vi "Reset layer template selection.vi"(7 "Force reset? (T)":bool=TRUE, 8 "error in (no error)":errorcluster, 11 "Data in":T1={"Class"={"Ants"=refnum, "Layer"=refnum, "Templates"=refnum, "Icon"=refnum, "Glyph"=refnum, "Settings"=refnum, "Tools"=refnum}, "Ref"={"Add Layer"=refnum, "Remove Layer"=refnum, "Line Text"=[], "Body Text Spec"=refnum, "DNL_Font"=refnum, "glyph path str"=refnum, "templates path str"=refnum, "Arrow Up"=refnum, "Arrow Down"=refnum, "IE VI Ref"=refnum, "Glyphs tree"=refnum, "Templates tree"=refnum, "Layer Icon Text"=refnum, "Layer Template"=refnum, "Clipboard"=refnum, "BW icon in"=refnum, "Color icon in"=refnum, "Layer Clust"=refnum, "Body Text"=refnum, "DNL_Framework Templates"=refnum, "Search Templates"=refnum, "TextMarker"=refnum, "Tab Control"=refnum, "Search Glyphs"=refnum, "Line Color"=refnum, "DNL_Glyphs []"=refnum, "Fill Color"=refnum, "Tools"=refnum, "Glyphs tree"=refnum, "Icon"=refnum, "Preview"=refnum, "Ants"=refnum, "Terminals"=refnum, "menu reference"=refnum, "LayerNames"=[], "GlyphLoadAnimation"=refnum, "TemplateLoadAnimation"=refnum, "refreshGlyphs"=refnum, "refreshTemplates"=refnum}, "Support"={"AntsRect"={"left"=0, "top"=0, "right"=0, "bottom"=0}, "Mouse Move Coords"={"Horizontal"=0, "Vertical"=0}, "Mouse Down Coords"={"Horizontal"=0, "Vertical"=0}, "Temp Coord"={"Horizontal"=0, "Vertical"=0}, "Action"=enum."Default", "Edge Color"=4914962, "Fill Color"=16860, "Mouse Down?"=FALSE, "Draft Mode?"=FALSE, "Temp Icon"=bytes[3102], "CTRL Pressed"=FALSE, "Move Selection?"=FALSE, "AntsRect Orig"={"left"=0, "top"=0, "right"=0, "bottom"=0}, "Text"="", "TM Set?"=FALSE, "Mouse inside icon?"=FALSE, "Tool (old value)"=0, "Pencil Move Color"=0, "Swap Colors?"=FALSE, "Shift pressed?"=FALSE}}) -> (0 "error out":errorcluster, 2 "Active Data []":i32[](array[numeric]), 3 "Data out":T1={"Class"={"Ants"=refnum, "Layer"=refnum, "Templates"=refnum, "Icon"=refnum, "Glyph"=refnum, "Settings"=refnum, "Tools"=refnum}, "Ref"={"Add Layer"=refnum, "Remove Layer"=refnum, "Line Text"=[], "Body Text Spec"=refnum, "DNL_Font"=refnum, "glyph path str"=refnum, "templates path str"=refnum, "Arrow Up"=refnum, "Arrow Down"=refnum, "IE VI Ref"=refnum, "Glyphs tree"=refnum, "Templates tree"=refnum, "Layer Icon Text"=refnum, "Layer Template"=refnum, "Clipboard"=refnum, "BW icon in"=refnum, "Color icon in"=refnum, "Layer Clust"=refnum, "Body Text"=refnum, "DNL_Framework Templates"=refnum, "Search Templates"=refnum, "TextMarker"=refnum, "Tab Control"=refnum, "Search Glyphs"=refnum, "Line Color"=refnum, "DNL_Glyphs []"=refnum, "Fill Color"=refnum, "Tools"=refnum, "Glyphs tree"=refnum, "Icon"=refnum, "Preview"=refnum, "Ants"=refnum, "Terminals"=refnum, "menu reference"=refnum, "LayerNames"=[], "GlyphLoadAnimation"=refnum, "TemplateLoadAnimation"=refnum, "refreshGlyphs"=refnum, "refreshTemplates"=refnum}, "Support"={"AntsRect"={"left"=0, "top"=0, "right"=0, "bottom"=0}, "Mouse Move Coords"={"Horizontal"=0, "Vertical"=0}, "Mouse Down Coords"={"Horizontal"=0, "Vertical"=0}, "Temp Coord"={"Horizontal"=0, "Vertical"=0}, "Action"=enum."Default", "Edge Color"=4914962, "Fill Color"=16860, "Mouse Down?"=FALSE, "Draft Mode?"=FALSE, "Temp Icon"=bytes[3102], "CTRL Pressed"=FALSE, "Move Selection?"=FALSE, "AntsRect Orig"={"left"=0, "top"=0, "right"=0, "bottom"=0}, "Text"="", "TM Set?"=FALSE, "Mouse inside icon?"=FALSE, "Tool (old value)"=0, "Pencil Move Color"=0, "Swap Colors?"=FALSE, "Shift pressed?"=FALSE}}, 5 "Layers selected?":bool)   [LabVIEW 2021]
uses:
  Controls/IE Data.ctl
  Class/Ants/Ants.lvclass
  Class/FakedArray/FakedArray.lvclass
  vi.lib/LabVIEW Icon API/lv_icon/Classes/Icon/Icon.lvclass
  Class/Icon Library/Glyph.lvclass
  Class/Settings/Settings.lvclass
  Class/Tools/Tools Paint.lvclass
  Controls/IE Classes.ctl
  Controls/References Cluster.ctl
  Controls/SupportClass.ctl
  <vilib>/Utility/miscctls.llb/LVPoint32TypeDef.ctl
  Controls/SupportClass_Action.ctl
  vi.lib/LabVIEW Icon API/lv_icon/Controls/IEColor.ctl
  Global Variables/Data.vi
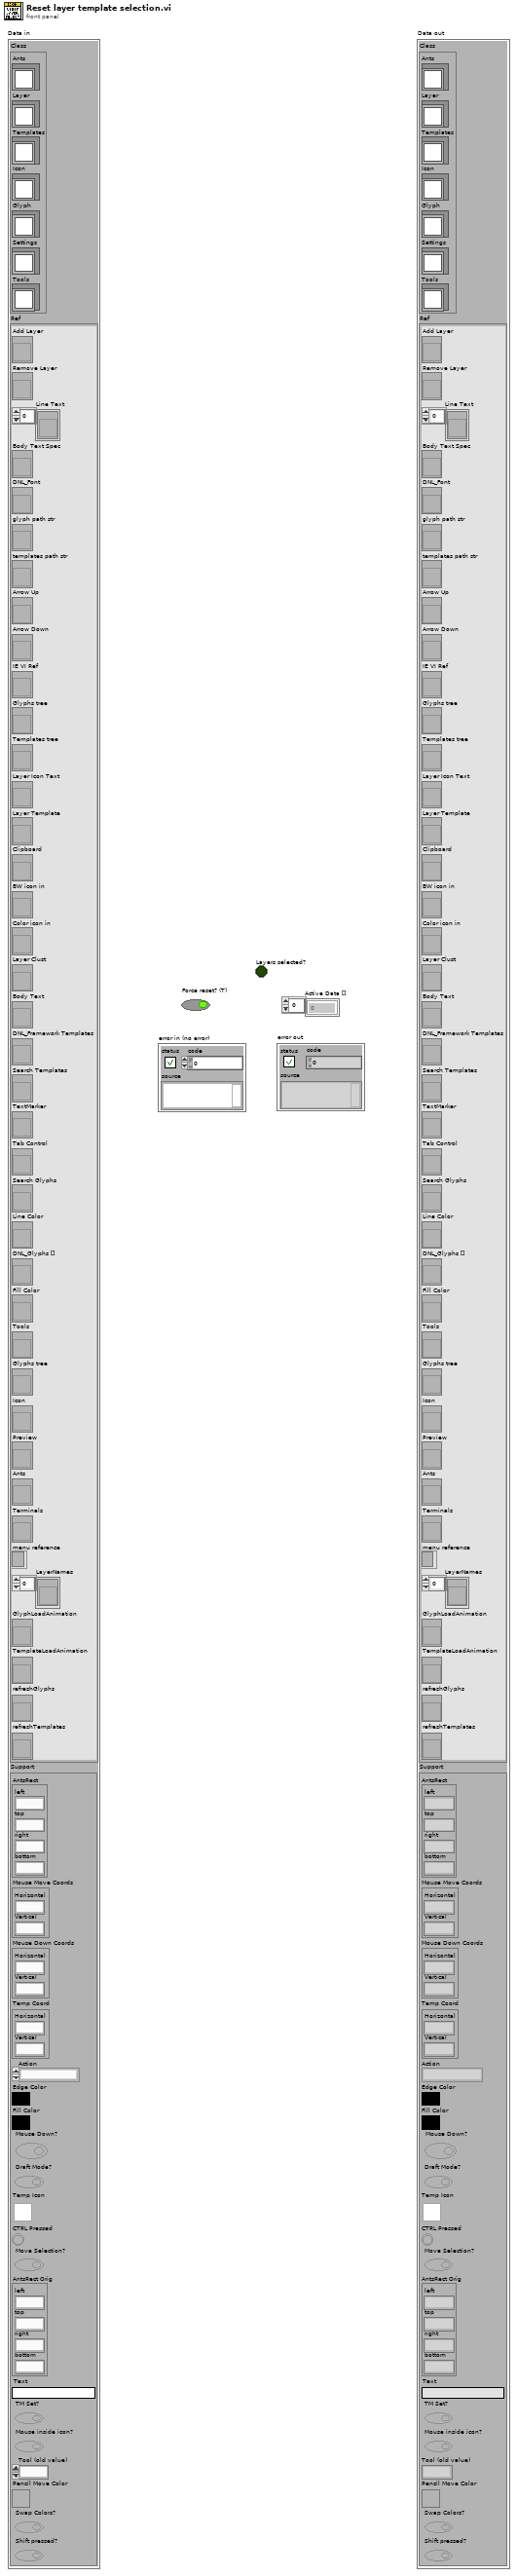
[diagram p1: front panel]
types:
  T1 = typedef "IE Data.ctl" = cluster{"Class":T2, "Ref":T3, "Support":T4}
  T2 = typedef "IE Classes.ctl" = cluster{"Ants":refnum<class "Ants.lvclass">, "Layer":refnum<class "FakedArray.lvclass">, "Templates":refnum<class "FakedArray.lvclass">, "Icon":refnum<class "Icon.lvclass">, "Glyph":refnum<class "Glyph.lvclass">, "Settings":refnum<class "Settings.lvclass">, "Tools":refnum<class "Tools Paint.lvclass">}
  T3 = typedef "References Cluster.ctl" = cluster{"Add Layer":refnum<vi>, "Remove Layer":refnum<vi>, "Line Text":refnum<vi>[], "Body Text Spec":refnum<vi>, "DNL_Font":refnum<vi>, "glyph path str":refnum<vi>, "templates path str":refnum<vi>, "Arrow Up":refnum<vi>, "Arrow Down":refnum<vi>, "IE VI Ref":refnum<vi>, "Glyphs tree":refnum<vi>, "Templates tree":refnum<vi>, "Layer Icon Text":refnum<vi>, "Layer Template":refnum<vi>, "Clipboard":refnum<vi>, "BW icon in":refnum<vi>, "Color icon in":refnum<vi>, "Layer Clust":refnum<vi>, "Body Text":refnum<vi>, "DNL_Framework Templates":refnum<vi>, "Search Templates":refnum<vi>, "TextMarker":refnum<vi>, "Tab Control":refnum<vi>, "Search Glyphs":refnum<vi>, "Line Color":refnum<vi>, "DNL_Glyphs []":refnum<vi>, "Fill Color":refnum<vi>, "Tools":refnum<vi>, "Glyphs tree":refnum<vi>, "Icon":refnum<vi>, "Preview":refnum<vi>, "Ants":refnum<vi>, "Terminals":refnum<vi>, "menu reference":refnum<k9>, "LayerNames":refnum<vi>[], "GlyphLoadAnimation":refnum<vi>, "TemplateLoadAnimation":refnum<vi>, "refreshGlyphs":refnum<vi>, "refreshTemplates":refnum<vi>}
  T4 = typedef "SupportClass.ctl" = cluster{"AntsRect":cluster{"left":i16, "top":i16, "right":i16, "bottom":i16}, "Mouse Move Coords":T5, "Mouse Down Coords":T5, "Temp Coord":T5, "Action":T6, "Edge Color":T7, "Fill Color":T7, "Mouse Down?":bool, "Draft Mode?":bool, "Temp Icon":picture, "CTRL Pressed":bool, "Move Selection?":bool, "AntsRect Orig":cluster{"left":i16, "top":i16, "right":i16, "bottom":i16}, "Text":string, "TM Set?":bool, "Mouse inside icon?":bool, "Tool (old value)":u32, "Pencil Move Color":u32, "Swap Colors?":bool, "Shift pressed?":bool}
  T5 = typedef "LVPoint32TypeDef.ctl" = cluster{"Horizontal":i32, "Vertical":i32}
  T6 = typedef "SupportClass_Action.ctl" = enum16{"Default", "Move Selection", "Glyph Library", "Tool"}
  T7 = typedef "IEColor.ctl" = u32
  T8 = cluster{"Minimum # of selected elements":u32, "Maximum # of selected elements":u32, "# Rows":u32, "# Cols":u32}
  T9 = cluster{"left":i16, "top":i16, "right":i16, "bottom":i16}
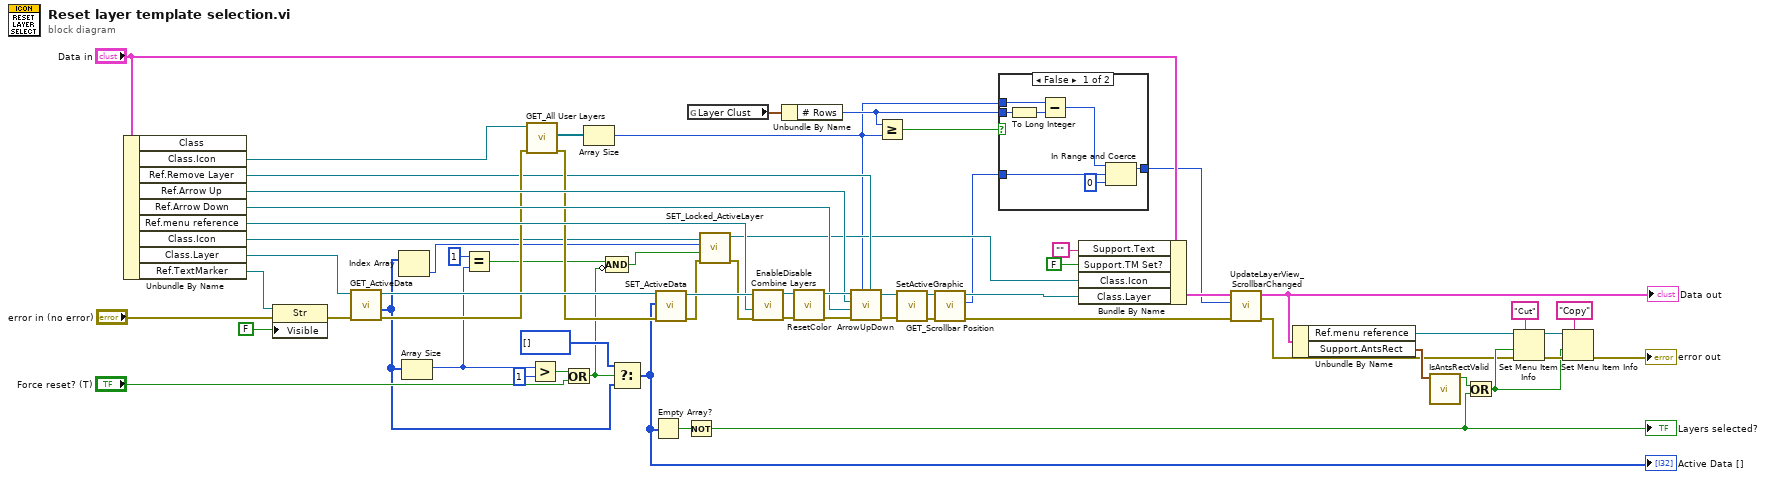
[diagram p0: block diagram]
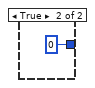
[diagram p2: hidden frame]
diagram:
  n1 = Unbundle By Name("Data in") -> ("Class.Icon"=w43:refnum<class "Icon.lvclass">, "Ref.Remove Layer"=w41:refnum<vi>, "Ref.Arrow Up"=w46:refnum<vi>, "Ref.Arrow Down"=w47:refnum<vi>, "Ref.menu reference"=w52:refnum<k9>, "Class.Icon"=w32:refnum<class "Icon.lvclass">, "Class.Layer"=w54:refnum<class "FakedArray.lvclass">, "Ref.TextMarker"=w2:refnum<vi>)  [unwired: 1 out]
  n2 = property class="Str"(reference=w2, error in="error in (no error)", "Visible"=FALSE) -> (error out=w3:errorcluster)  [unwired: 1 out]
  n3 = call-dynamic "GET_ActiveData.vi"("error in (no error)"=w3, "FakedArray in"=w54) -> ("error out"=w45:errorcluster, "Active Data []"=w23:i32[], "FakedArray out"=w61:refnum<class "FakedArray.lvclass">)  [unwired: 7 out]
  n4 = Index Array(array=w23) -> (element=w22:i32)  [unwired: 1 in]
  n5 = Array Size(array=w23) -> (size(s)=w29:i32)
  n6 = Equal?(x=1, y=w29) -> (x = y?=w26:bool)
  n7 = call-dynamic "GET_All User Layers.vi"("error in (no error)"=w45, "Icon.lvclass in"=w43) -> ("error out"=w44:errorcluster, "User Layer"=w42:refnum<class "Layer.lvclass">[])  [unwired: 8 out]
  n8 = Greater?(x=w29, y=1) -> (0:w31:bool)
  n9 = Or(x=w31, y="Force reset? (T)") -> (x .or. y?=w30:bool)
  n10 = Array Size(array=w42) -> (size(s)=w8:i32)
  n11 = Compound Arithmetic op=AND(w26, invert w30) -> (w27:bool)
  n12 = Select(t=i32[] [], s=w30, f=w23) -> (s? t:f=w6:i32[])
  "Active Data []" <- w6
  n13 = Empty Array?(array=w6) -> (empty?=w60:bool)
  n14 = call-dynamic "SET_ActiveData.vi"("error in (no error)"=w44, "Active Data"=w6, "FakedArray.lvclass in"=w61) -> ("error out"=w25:errorcluster, "FakedArray.lvclass out"=w64:refnum<class "FakedArray.lvclass">)  [unwired: 7 out]
  n15 = Not(x=w60) -> (.not. x?=w7:bool)
  "Layers selected?" <- w7
  n16 = global read "Data.vi" "Layer Clust"() -> (w12:T8)
  n17 = call-dynamic "SET_Locked_ActiveLayer.vi"("error in (no error)"=w25, "Layers Locked?"=w27, "Active Layer"=w22, "Icon.lvclass in"=w32) -> ("error out"=w24:errorcluster, "Icon.lvclass out"=w21:refnum<class "Icon.lvclass">)  [unwired: 6 in]
  n18 = call "EnableDisable Combine Layers.vi"("error in"=w24, "menu reference"=w52, "Layers Cluster"=w64) -> ("error out"=w63:errorcluster, "FakedArray out"=w62:refnum<class "FakedArray.lvclass">)  [unwired: 1 in, 6 out]
  n19 = Unbundle By Name(w12) -> ("# Rows"=w9:u32)
  n20 = call "ResetColor.vi"("error in (no error)"=w63, "FakedArray in"=w62) -> ("error out"=w50:errorcluster, "FakedArray out"=w51:refnum<class "FakedArray.lvclass">)  [unwired: 8 out]
  n21 = call "ArrowUpDown.vi"("Remove Layer"=w41, "# Layers"=w8, "error in (no error)"=w50, "Arrow Down"=w47, "Arrow Up"=w46, "FakedArray in"=w51) -> ("error out"=w49:errorcluster, "FakedArray out"=w48:refnum<class "FakedArray.lvclass">)  [unwired: 4 out]
  n22 = Greater Or Equal?(x=w9, y=w8) -> (x >= y?=w11:bool)
  n23 = call-dynamic "SetActiveGraphic.vi"("error in (no error)"=w49, "FakedArray in"=w48) -> ("error out"=w15:errorcluster, "FakedArray out"=w17:refnum<class "FakedArray.lvclass">)  [unwired: 4 in, 4 out]
  n24 = call-dynamic "GET_Scrollbar Position.vi"("error in (no error)"=w15, "FakedArray.lvclass in"=w17) -> ("error out"=w14:errorcluster, "Scrollbar Position"=w10:i32, "FakedArray.lvclass out"=w16:refnum<class "FakedArray.lvclass">)  [unwired: 7 in]
  n25 = case shown="False" w11 {
    tunnel: [w70 0 ("lower limit")] -> w13
    tunnel: w10 -> [w66 _]
    tunnel: w9 -> [w69 _]
    tunnel: w8 -> [w68 _]
    frame False {
      n26 = To Long Integer(number=w69) -> (32bit integer=w65:i32)
      n27 = Subtract(x=w68, y=w65) -> (x-y=w67:i32)
      n28 = In Range and Coerce(upper limit=w67, x=w66, lower limit=0) -> (coerced(x)=w70:i32)  [unwired: 1 out]
    }
    frame True {
    }
  }
  n29 = Bundle By Name(cluster="Data in", "Support.Text"="", "Support.TM Set?"=FALSE, "Class.Icon"=w21, "Class.Layer"=w16) -> (w20:T1)
  n30 = call "UpdateLayerView_ScrollbarChanged.vi"("error in"=w14, "Scrollbar Position"=w13, "Data in"=w20) -> ("error out"=w18:errorcluster, "Data out"=w19:T1)  [unwired: 7 out]
  "Data out" <- w19
  n31 = Unbundle By Name(w19) -> ("Ref.menu reference"=w40:refnum<k9>, "Support.AntsRect"=w35:T9)
  n32 = call "IsAntsRectValid.vi"("AntsRect"=w35) -> ("Valid?"=w33:bool)  [unwired: 10 out]
  n33 = Or(x=w33, y=w7) -> (x .or. y?=w34:bool)
  n34 = Set Menu Item Info(7:"Cut" ("item tag"), 8:w18, 9:w34, 11:w40) -> (0:w39:errorcluster, 3:w37:refnum<k9>)  [unwired: 3 out]
  n35 = Set Menu Item Info(7:"Copy" ("item tag"), 8:w39, 9:w34, 11:w37) -> (0:→"error out":errorcluster)  [unwired: 4 out]
